vi "workbook read only recommended.vi"(8 "error in (no error)":errorcluster, 11 "workbook":u32) -> (0 "error out":errorcluster)   [LabVIEW 8.6]
doc: "void workbook_read_only_recommended(lxw_workbook workbook);"
uses:
  pending_lvxlsxwriter/xlsxwriter.dll
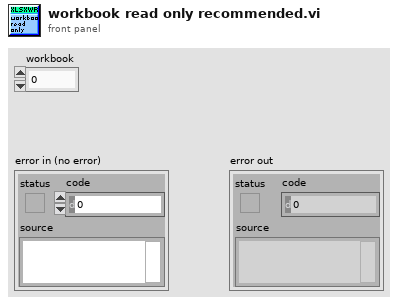
[diagram p1: front panel]
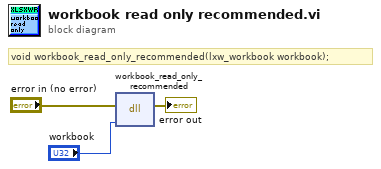
[diagram p0: block diagram]
diagram:
  # "void workbook_read_only_recommended(lxw_workbook workbook);"
  n1 = dll-call lib="C:/Users/WDAGUtilityAccount/Desktop/pending_lvxlsxwriter/xlsxwriter.*" fn="workbook_read_only_recommended"(error in="error in (no error)", "workbook"="workbook") -> (error out=→"error out":errorcluster)  [unwired: 4 in, 1 out]
